vi "polling_events.vi"() -> ()   [LabVIEW 2010]
uses:
  socket_type.ctl
  socket_options.ctl
  zmq_context.lvclass
  zeromq.lvlib
  zmq_socket.lvclass
panel:
  out "messages":string[](array[string])
  in  "endpoint":string="tcp://127.0.0.1:5555"
  # "ZeroMQ polling-based receive events"
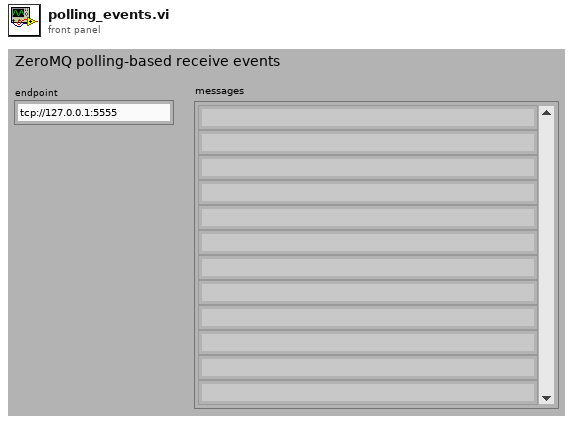
[diagram p1: front panel]
types:
  T1 = typedef "zeromq.lvlib/socket_options.ctl" = enum8{"NONE", "ZMQ_HWM", "<2>", "ZMQ_SWAP", "ZMQ_AFFINITY", "ZMQ_IDENTITY", "ZMQ_SUBSCRIBE", "ZMQ_UNSUBSCRIBE", "ZMQ_RATE", "ZMQ_RECOVERY_IVL", "ZMQ_MCAST_LOOP", "ZMQ_SNDBUF", "ZMQ_RCVBUF", "ZMQ_RCVMORE", "ZMQ_FD", "ZMQ_EVENTS", "ZMQ_TYPE", "ZMQ_LINGER", "ZMQ_RECONNECT_IVL", "ZMQ_BACKLOG", "ZMQ_RECOVERY_IVL_MSEC", "ZMQ_RECONNECT_IVL_MAX", "ZMQ_MAXMSGSIZE", "ZMQ_SNDHWM", "ZMQ_RCVHWM", "ZMQ_MULTICAST_HOPS", "<26>", "ZMQ_RCVTIMEO", "ZMQ_SNDTIMEO", "<29>", "<30>", "ZMQ_IPV4ONLY", "ZMQ_LAST_ENDPOINT", "ZMQ_ROUTER_MANDATORY", "ZMQ_TCP_KEEPALIVE", "ZMQ_TCP_KEEPALIVE_CNT", "ZMQ_TCP_KEEPALIVE_IDLE", "ZMQ_TCP_KEEPALIVE_INTVL", "ZMQ_TCP_ACCEPT_FILTER", "ZMQ_DELAY_ATTACH_ON_CONNECT", "ZMQ_XPUB_VERBOSE"}
  T2 = typedef "zeromq.lvlib/socket_type.ctl" = enum8{"ZMQ_PAIR", "ZMQ_PUB", "ZMQ_SUB", "ZMQ_REQ", "ZMQ_REP", "ZMQ_DEALER", "ZMQ_ROUTER", "ZMQ_PULL", "ZMQ_PUSH", "ZMQ_XPUB", "ZMQ_XSUB"}
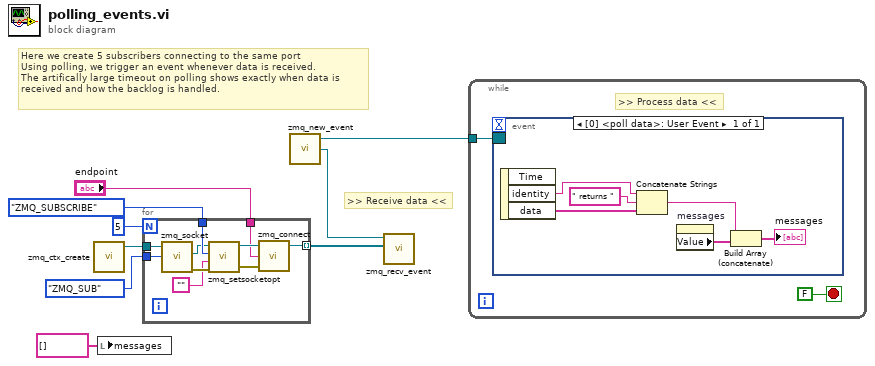
[diagram p0: block diagram]
diagram:
  # "Here we create 5 subscribers connecting to the same port\nUsing polling, we trigger an event whenever data is received.\nThe artifically large timeout on polling shows exactly when data is\nreceived and how the backlog is handled."
  # ">> Receive data <<"
  n1 = call "zmq_ctx_create.vi"() -> ("context out"=w9:refnum<class "zmq_context.lvclass">)  [unwired: 4 in, 1 out]
  n2 = local write "messages"(string[] [] ("messages")) -> ()
  n3 = for {
    N: 5 -> [_]
    tunnel: w9 -> [w19]
    tunnel: [w18] -> w3 mode=indexing
    tunnel: socket_options."ZMQ_SUBSCRIBE" ("option") -> [w16]
    tunnel: socket_type."ZMQ_SUB" ("socket type") -> [w15]
    tunnel: "endpoint" -> [w11]
    n4 = call "zmq_socket.vi"("socket type"=w15, "context in"=w19) -> ("error out"=w17:errorcluster, "socket out"=w10:refnum<class "zmq_socket.lvclass">)  [unwired: 3 in, 1 out]
    n5 = call "zmq_setsocketopt.vi"("error in"=w17, "value"="", "option"=w16, "socket in"=w10) -> ("error out"=w12:errorcluster, "socket out"=w13:refnum<class "zmq_socket.lvclass">)  [unwired: 2 in]
    n6 = call "zmq_connect.vi"("error in"=w12, "endpoint"=w11, "socket in"=w13) -> ("socket out"=w18:refnum<class "zmq_socket.lvclass">)  [unwired: 1 in, 1 out]
  }
  n7 = call "zmq_new_event.vi"() -> ("user event"=w1:refnum<user-event>, "event ref out"=w2:refnum<event-registration>)  [unwired: 3 in, 1 out]
  n8 = call "zmq_recv_event.vi"("sockets"=w3, "poll event"=w1) -> ()  [unwired: 4 in, 2 out]
  n9 = while {
    tunnel: w2 -> [w21]
    stop <- FALSE stop-if-true
    # ">> Process data <<"
    n10 = event shown="[0] <poll data>: User Event" {
      selector: w21 -> [_]
      dyn-events: _ -> [_]
      timeout: _ -> [_]
      event User Event {
        n11 = event-data() -> ("identity"=w22:string, "data"=w23:string[])  [unwired: 1 in, 1 out]
        n12 = Concatenate Strings(w22, " returns " ("string"), w23) -> (w26:string)
        n13 = property on="messages" class="Arr (strict)"() -> ("Value"=w25:string[])  [unwired: 2 in, 2 out]
        n14 = Build Array (concatenate)(w26, w25) -> (→"messages":string[])
      }
    }
  }
